vi "PC_Main_SequenceEditor.vi"() -> ()   [LabVIEW 2010]
uses:
  Ctls/StepData.ctl
  <vilib>/Utility/error.llb/DialogType.ctl
  <vilib>/Pansino Software/LabVIEW Architecture/PSARC_Queue Management.llb/PSARC_Queue Create_Single.vi
  <vilib>/Pansino Software/LabVIEW Architecture/PSARC_Queue Management.llb/PSARC_Queue Destroy_Single.vi
  <vilib>/Pansino Software/LabVIEW Architecture/PSARC_Queue Management.llb/PSARC_Queue Valid.vi
  <vilib>/Pansino Software/LabVIEW Architecture/PSARC_Queue Management.llb/PSARC_Queue Insert Element.vi
  <vilib>/Pansino Software/LabVIEW Architecture/PSARC_Queue Management.llb/PSARC_Queue Remove Element.vi
  PC_DynVIs/PC_CallRTGuidedMunitions.vi
panel:
  in  "new element/subarray":T1
  out "Error Report 2":string
  out "Current State 2":string
  in  "TempVariable":T2
  in  "New":bool
  in  "Load":bool
  in  "Save":bool
  in  "Run":bool
  in  "DeleteStep":bool
  in  "EditStep":bool
  in  "AddStep":bool
  in  "Multicolumn Listbox":i32(listbox)
  out "Error Report":string
  out "Current State":string
  in  "OK":bool
  in  "Exit Program":bool
  # "————————————————\nYou could add your temporary variables\nhere.\nThis Control should be saved as a\nvi in your project folder,The proposed vi's block diagram is shown in the picture\n\n\n\n\n\n\n\n————————————————"
  # "/* Path */\nYou could add your path here."
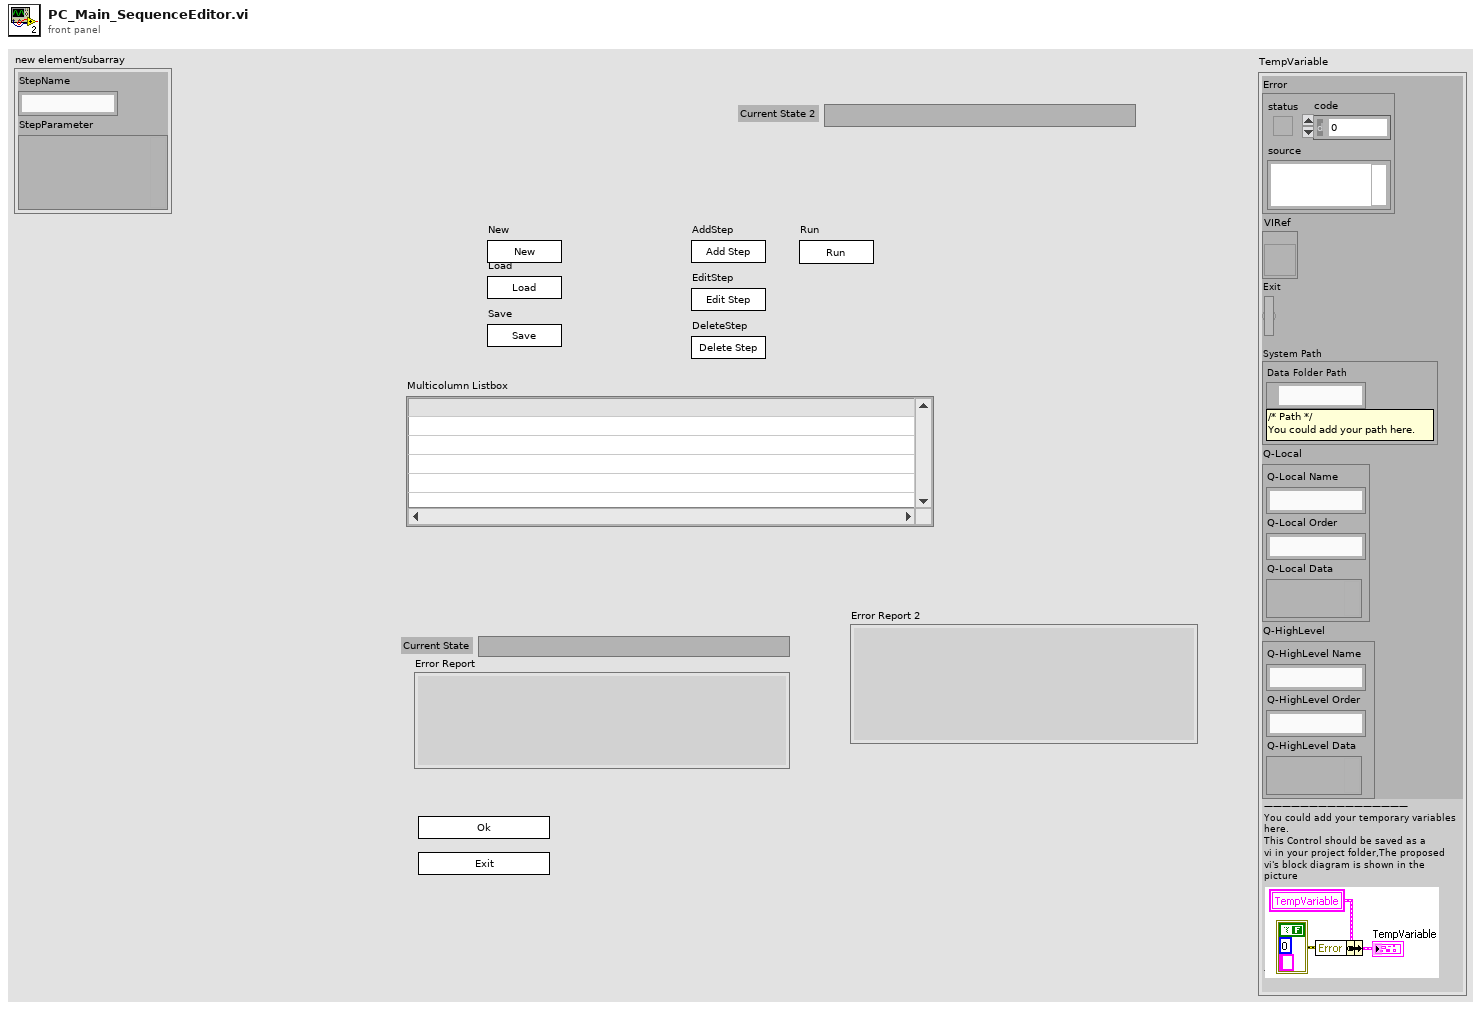
[diagram p1: front panel]
types:
  T1 = typedef "StepData.ctl" = cluster{"StepName":string, "StepParameter":variant}
  T2 = cluster{"Error":errorcluster, "VIRef":refnum<vi>, "Exit":bool, "System Path":cluster{"Data Folder Path":path}, "Q-Local":cluster{"Q-Local Name":string, "Q-Local Order":string, "Q-Local Data":variant}, "Q-HighLevel":cluster{"Q-HighLevel Name":string, "Q-HighLevel Order":string, "Q-HighLevel Data":variant}}
  T3 = typedef "PC_Main_SequenceEditor_TempVariable.ctl" = cluster{"Error":errorcluster, "Event":string, "Data":variant, "VIRef":refnum<vi>, "Exit":bool, "Main Q-Array":string, "Sequence":T1[]}
  T4 = typedef "DialogType.ctl" = u16
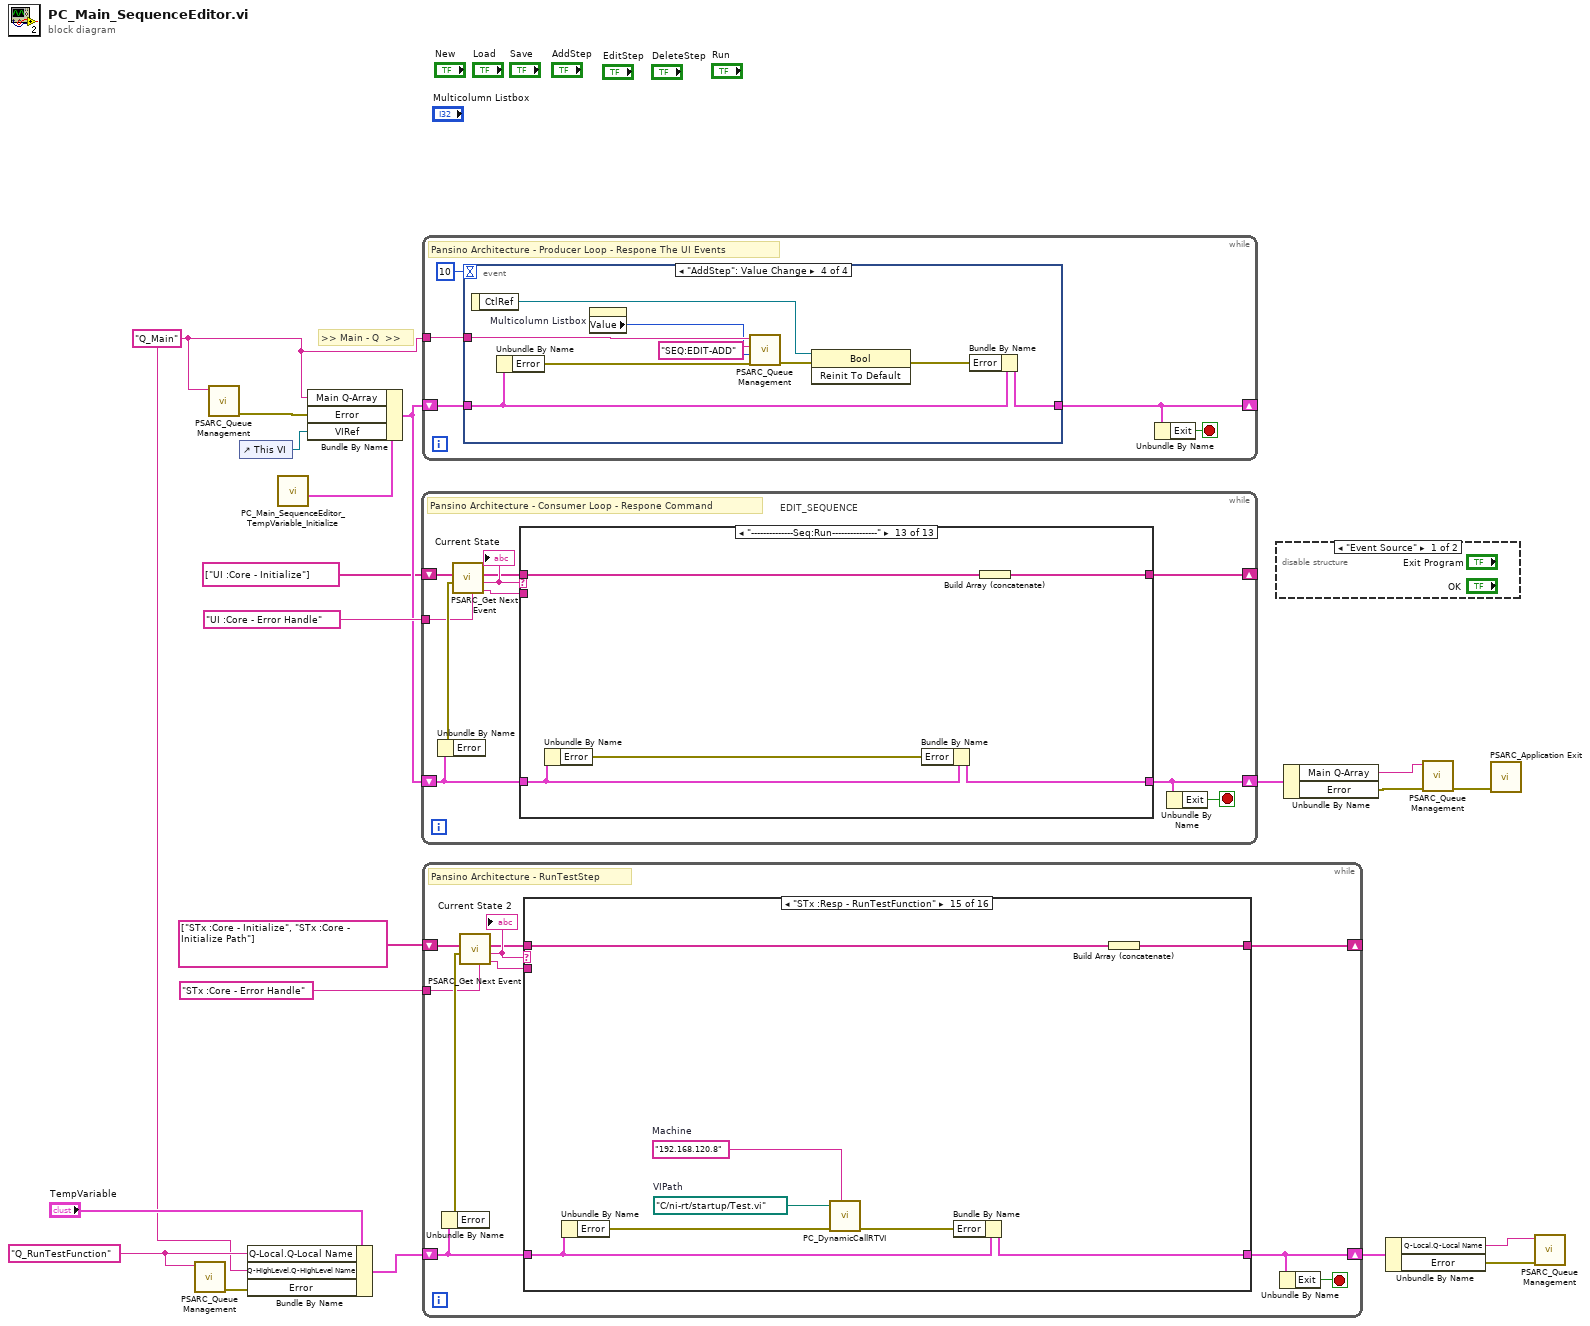
[diagram p0: block diagram]
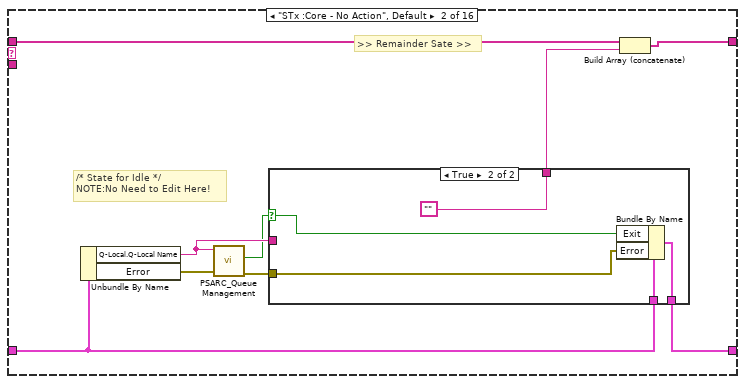
[diagram p3: hidden frame]
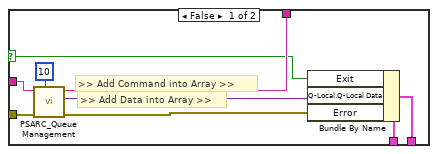
[diagram p4: hidden frame]
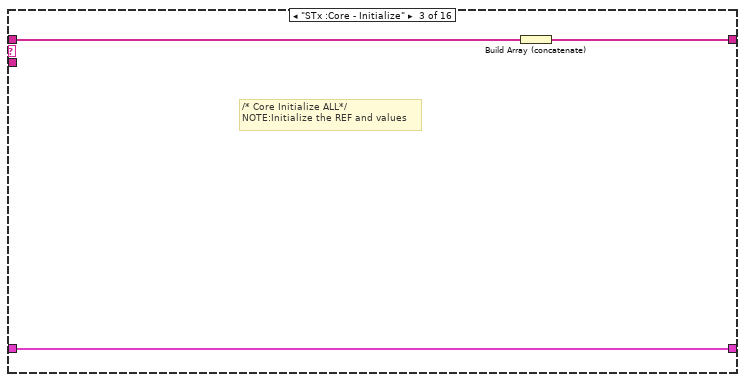
[diagram p5: hidden frame]
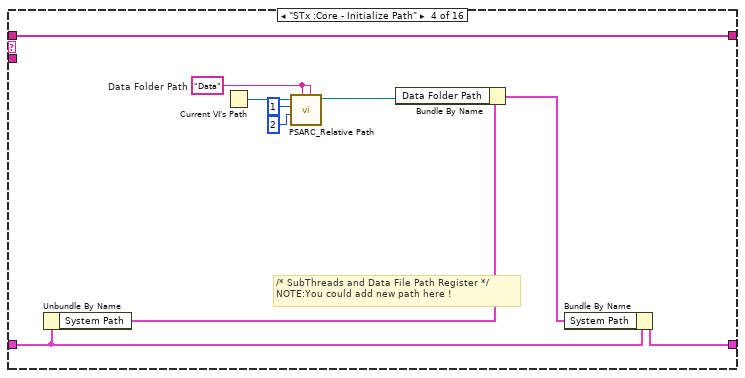
[diagram p6: hidden frame]
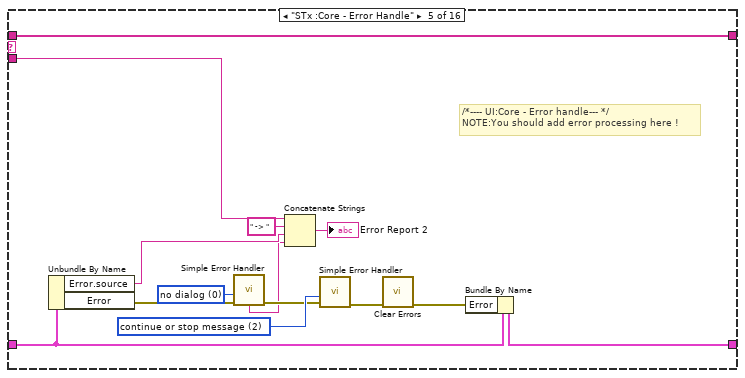
[diagram p7: hidden frame]
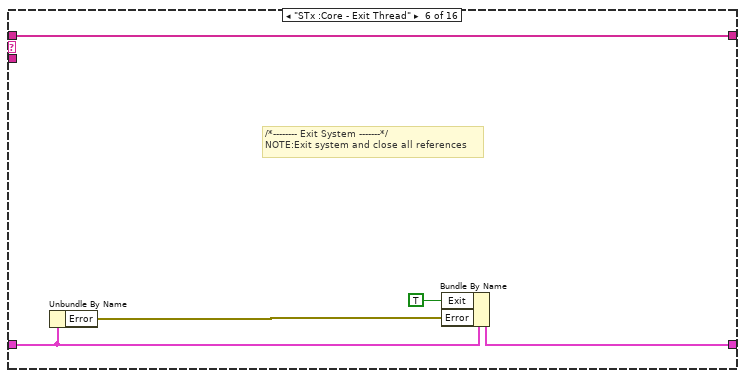
[diagram p8: hidden frame]
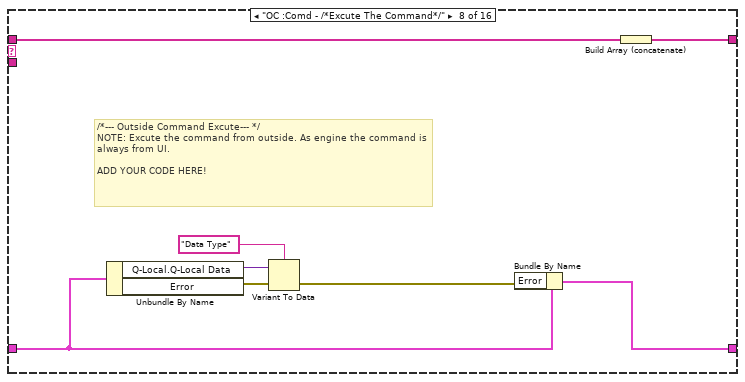
[diagram p10: hidden frame]
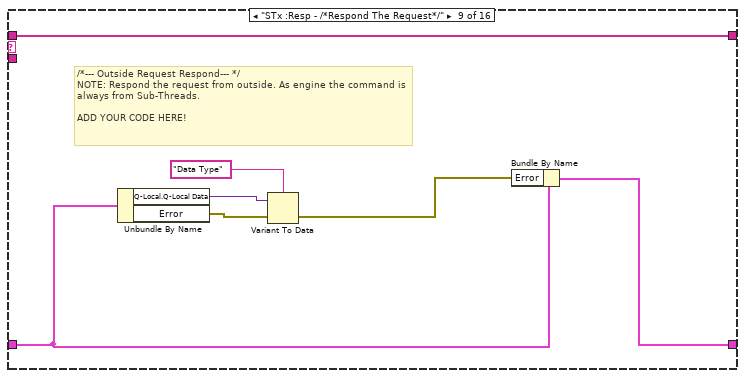
[diagram p11: hidden frame]
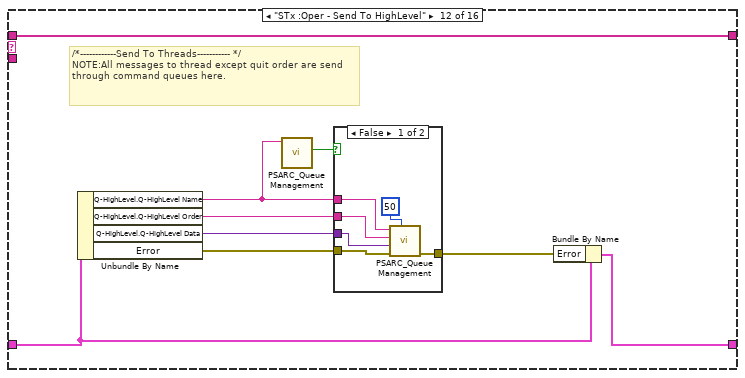
[diagram p14: hidden frame]
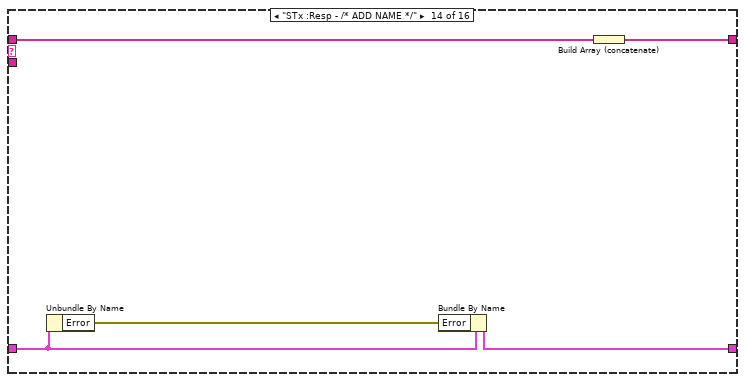
[diagram p17: hidden frame]
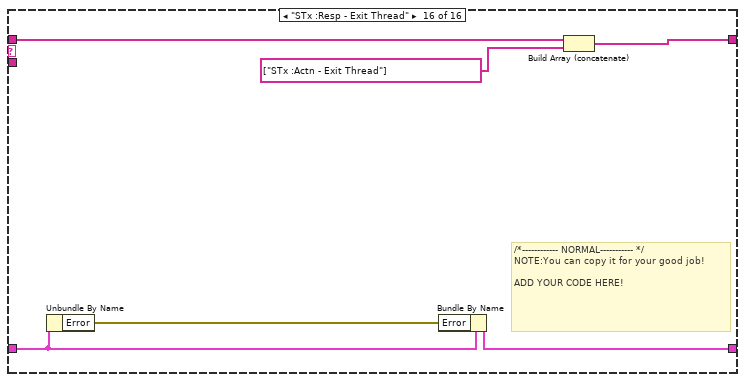
[diagram p18: hidden frame]
diagram:
  w2 = "Q_RunTestFunction" ("Queue Name")
  w1 = "Q_Main" ("Queue name(unamed)")
  # ">> Main - Q  >>"
  n1 = call-poly <vilib>:"PSARC_Queue Management.vi"("Queue Name"=w2) -> ("error out"=w10:errorcluster)  [unwired: 9 in, 1 out]
  n2 = call-poly <vilib>:"PSARC_Queue Management.vi"("Queue Name"=w1) -> ("error out"=w17:errorcluster)  [unwired: 9 in, 1 out]
  n3 = control-ref of="This VI"() -> (w18:refnum<vi>)
  n4 = Bundle By Name(cluster="TempVariable", "Q-Local.Q-Local Name"=w2, "Q-HighLevel.Q-HighLevel Name"=w1, "Error"=w10) -> (w6:T2)
  n5 = call "PC_Main_SequenceEditor_TempVariable_Initialize.vi"() -> ("TempVariable"=w11:T3)  [unwired: 11 in]
  n6 = Bundle By Name(cluster=w11, "Main Q-Array"=w1, "Error"=w17, "VIRef"=w18) -> (w19:T3)
  n7 = while {
    shift-right: [w24] -> w13
    shift-left: w19 -> [w26]
    shift-right: [w27] -> _
    shift-left: string[] ["UI :Core - Initialize"] -> [w30]
    tunnel: "UI :Core - Error Handle" ("Error Handle") -> [w22]
    stop <- w23 stop-if-true
    # "EDIT_SEQUENCE"
    # "Pansino Architecture - Consumer Loop - Respone Command"
    n8 = Unbundle By Name(w26) -> ("Error"=w25:errorcluster)
    n9 = call <vilib>:"PSARC_Get Next Event.vi"("Error Handle"=w22, "error in (no error)"=w25, "event queue in"=w30) -> ("prev event"=w21:string, "next event"=w29:string, "event queue out"=w28:string[])  [unwired: 3 in]
    "Current State" <- w29
    n10 = case shown="\"--------------Seq:Run---------------\"" w29 {
      tunnel: w26 -> [w31 w40 w55 w58 w61 w65 w70 w76 w81 w92 w97 w102 w107]
      tunnel: w28 -> [w32 w38 w57 w59 w64 w66 w68 w74 w79 w90 w95 w100 w105]
      tunnel: [w32 w37 w57 w59 w64 w66 w67 w73 w78 w89 w94 w99 w104] -> w27
      tunnel: [w31 w39 w56 w58 w62 w65 w69 w75 w80 w91 w96 w101 w106] -> w24
      tunnel: w21 -> [_ _ w45 _ _ _ _ _ _ _ _ _ _]
      frame "----------Core Status----------" {
      }
      frame "UI :Core - No Action", Default {
        # "/* State for Idle */\nNo Need to Edit here!"
        # ">> Add Data into the Array >>"
        # ">> Add Command into the Array >>"
        # ">> Remainder Sate >>"
        n11 = Unbundle By Name(w40) -> ("Main Q-Array"=w34:string, "Error"=w41:errorcluster)
        n12 = call-poly <vilib>:"PSARC_Queue Management.vi"("Time out(-1)_queue out"=10, "error in (no error)"=w41, "Queue Name(unamed)"=w34) -> ("error out"=w43:errorcluster, "Data"=w42:variant, "Event"=w35:string)  [unwired: 5 in, 1 out]
        n13 = Wait (ms)(milliseconds to wait=u32 50 ("等待时间（毫秒）")) -> ()  [unwired: 1 out]
        n14 = Bundle By Name(cluster=w40, "Data"=w42, "Error"=w43) -> (w39:T3)
        n15 = Build Array (concatenate)(w38, w35) -> (w37:string[])
      }
      frame "UI :Core - Error Handle" {
        w44 = T4 0 items=["no dialog", "OK message", "continue or stop message", "OK message + warnings", "continue/stop + warnings"] ("type of dialog (OK msg:1)")
        w52 = T4 2 items=["no dialog", "OK message", "continue or stop message", "OK message + warnings", "continue/stop + warnings"] ("type of dialog (OK msg:1)")
        n16 = Unbundle By Name(w55) -> ("Error.source"=w46:string, "Error"=w49:errorcluster)
        n17 = call <vilib>:"Simple Error Handler.vi"("type of dialog (OK msg:1)"=w44, "error in (no error)"=w49) -> ("error out"=w48:errorcluster, "message"=w47:string)  [unwired: 3 in, 3 out]
        n18 = Concatenate Strings(w45, " -> " ("字符串"), w46, w47) -> (→"Error Report":string)
        n19 = call <vilib>:"Simple Error Handler.vi"("type of dialog (OK msg:1)"=w52, "error in (no error)"=w48) -> ("error out"=w54:errorcluster)  [unwired: 3 in, 4 out]
        n20 = call <vilib>:"Clear Errors.vi"("error in (no error)"=w54) -> ("error out"=w53:errorcluster)  [unwired: 6 in]
        n21 = Bundle By Name(cluster=w55, "Error"=w53) -> (w56:T3)
      }
      frame "UI :Core - Initialize" {
        # "/* Resident Queues Register */\nNo Need to Edit here!"
      }
      frame "UI :Core - Exit System" {
        # "/*-------- Exit System -------*/\nExit system and close all references"
        n22 = Unbundle By Name(w61) -> ("Error"=w63:errorcluster)
        n23 = Bundle By Name(cluster=w61, "Exit"=TRUE, "Error"=w63) -> (w62:T3)
      }
      frame "----------Respond Events----------" {
      }
      frame "UI :Resp - /* ADD NAME */" {
        n24 = Unbundle By Name(w70) -> ("Error"=w71:errorcluster)
        n25 = Bundle By Name(cluster=w70, "Error"=w71) -> (w69:T3)
        n26 = Build Array (concatenate)(w68) -> (w67:string[])
      }
      frame "UI :Resp - Exit Event" {
        # "/*------------ NORMAL----------- */\nADD YOUR CODE HERE!\nNOTE:You can copy it for your good job!"
        n27 = Unbundle By Name(w76) -> ("Error"=w77:errorcluster)
        n28 = Bundle By Name(cluster=w76, "Error"=w77) -> (w75:T3)
        n29 = Build Array (concatenate)(w74, string[] ["UI :Core - Exit System"] ("数组")) -> (w73:string[])
      }
      frame "--------------Seq:Edit---------------" {
        n30 = Unbundle By Name(w81) -> ("Error"=w82:errorcluster)
        n31 = Bundle By Name(cluster=w81, "Error"=w82) -> (w80:T3)
        n32 = Build Array (concatenate)(w79) -> (w78:string[])
      }
      frame "SEQ:EDIT-ADD" {
        n33 = Unbundle By Name(w92) -> ("Data"=w84:variant, "Sequence"=w88:T1[], "Error"=w93:errorcluster)
        n34 = Variant To Data(Variant=w84, type=0 ("index")) -> (data=w83:i32)  [unwired: 1 in, 1 out]
        n35 = Insert Into Array(array=w88, index=w83, new element="new element/subarray") -> (w87:T1[])
        n36 = Bundle By Name(cluster=w92, "Sequence"=w87, "Error"=w93) -> (w91:T3)
        n37 = Build Array (concatenate)(w90) -> (w89:string[])
      }
      frame "SEQ:EDIT-EDIT" {
        n38 = Unbundle By Name(w97) -> ("Error"=w98:errorcluster)
        n39 = Bundle By Name(cluster=w97, "Error"=w98) -> (w96:T3)
        n40 = Build Array (concatenate)(w95) -> (w94:string[])
      }
      frame "SEQ:EDIT-DELETE" {
        n41 = Unbundle By Name(w102) -> ("Error"=w103:errorcluster)
        n42 = Bundle By Name(cluster=w102, "Error"=w103) -> (w101:T3)
        n43 = Build Array (concatenate)(w100) -> (w99:string[])
      }
      frame "--------------Seq:Run---------------" {
        n44 = Unbundle By Name(w107) -> ("Error"=w108:errorcluster)
        n45 = Bundle By Name(cluster=w107, "Error"=w108) -> (w106:T3)
        n46 = Build Array (concatenate)(w105) -> (w104:string[])
      }
    }
    n47 = Unbundle By Name(w24) -> ("Exit"=w23:bool)
  }
  n48 = while {
    shift-right: [w111] -> _
    shift-left: w19 -> [w112]
    tunnel: w1 -> [w109]
    stop <- w110 stop-if-true
    # "Pansino Architecture - Producer Loop - Respone The UI Events"
    n49 = event shown="[3] \"AddStep\": Value Change" {
      selector: _ -> [_ _ _ _]
      dyn-events: _ -> [_ _ _ _]
      timeout: 10 -> [_ _ _ _]
      tunnel: w112 -> [w117 w121 w126 w135]
      tunnel: [w116 w120 w125 w134] -> w111
      tunnel: w109 -> [w115 w118 w124 w133]
      event Timeout {
        n50 = event-data() -> ()  [unwired: 1 in, 1 out]
        n51 = call-poly <vilib>:"PSARC_Queue Management.vi"("Queue Name(unamed)"=w115) -> ("Not a queue?"=w114:bool)  [unwired: 9 in, 1 out]
        n52 = Bundle By Name(cluster=w117, "Exit"=w114) -> (w116:T3)
      }
      event "Exit Program": Value Change {
        n53 = event-data() -> ()  [unwired: 1 in, 1 out]
        n54 = Unbundle By Name(w121) -> ("Error"=w122:errorcluster)
        n55 = call-poly <vilib>:"PSARC_Queue Management.vi"("error in (no error)"=w122, "Event"="UI :Resp - Exit Event", "Queue Name(unamed)"=w118) -> ("error out"=w119:errorcluster)  [unwired: 7 in, 1 out]
        n56 = Bundle By Name(cluster=w121, "Error"=w119) -> (w120:T3)
      }
      event "OK": Value Change {
        n57 = event-data() -> ("CtlRef"=w131:refnum<vi>)  [unwired: 1 in]
        n58 = Unbundle By Name(w126) -> ("Error"=w129:errorcluster)
        n59 = call-poly <vilib>:"PSARC_Queue Management.vi"("error in (no error)"=w129, "Event"="UI :Resp - /* ADD NAME */", "Queue Name(unamed)"=w124) -> ("error out"=w128:errorcluster)  [unwired: 7 in, 1 out]
        n60 = invoke class="Bool" method="Reinit To Default"(reference=w131, error in=w128) -> (error out=w127:errorcluster)  [unwired: 1 in, 2 out]
        n61 = Bundle By Name(cluster=w126, "Error"=w127) -> (w125:T3)
      }
      event "AddStep": Value Change {
        n62 = event-data() -> ("CtlRef"=w140:refnum<vi>)  [unwired: 1 in]
        n63 = Unbundle By Name(w135) -> ("Error"=w138:errorcluster)
        n64 = property on="Multicolumn Listbox" class="MCListbox (strict)"() -> ("Value"=w132:i32)  [unwired: 2 in, 2 out]
        n65 = call-poly <vilib>:"PSARC_Queue Management.vi"("error in (no error)"=w138, "Data"=w132, "Event"="SEQ:EDIT-ADD", "Queue Name(unamed)"=w133) -> ("error out"=w137:errorcluster)  [unwired: 6 in, 1 out]
        n66 = invoke class="Bool" method="Reinit To Default"(reference=w140, error in=w137) -> (error out=w136:errorcluster)  [unwired: 1 in, 2 out]
        n67 = Bundle By Name(cluster=w135, "Error"=w136) -> (w134:T3)
      }
    }
    n68 = Unbundle By Name(w111) -> ("Exit"=w110:bool)
  }
  n69 = while {
    shift-right: [w144] -> w9
    shift-left: w6 -> [w146]
    shift-right: [w147] -> _
    shift-left: string[] ["STx :Core - Initialize", "STx :Core - Initialize Path"] -> [w150]
    tunnel: "STx :Core - Error Handle" ("Error Handle") -> [w142]
    stop <- w143 stop-if-true
    # "Pansino Architecture - RunTestStep"
    n70 = Unbundle By Name(w146) -> ("Error"=w145:errorcluster)
    n71 = call <vilib>:"PSARC_Get Next Event.vi"("Error Handle"=w142, "error in (no error)"=w145, "event queue in"=w150) -> ("prev event"=w141:string, "next event"=w149:string, "event queue out"=w148:string[])  [unwired: 3 in]
    "Current State 2" <- w149
    n72 = case shown="\"STx :Resp - RunTestFunction\"" w149 {
      tunnel: w146 -> [w151 w161 w177 w186 w200 w204 w208 w214 w223 w225 w227 w234 w245 w250 w259 w264]
      tunnel: w148 -> [w152 w159 w178 w188 w202 w207 w209 w217 w224 w226 w228 w237 w246 w248 w257 w262]
      tunnel: [w152 w158 w176 w188 w202 w207 w209 w215 w224 w226 w228 w237 w246 w247 w256 w261] -> w147
      tunnel: [w151 w160 w177 w187 w201 w205 w208 w216 w222 w225 w227 w233 w245 w249 w258 w263] -> w144
      tunnel: w141 -> [_ _ _ _ w193 _ _ _ _ _ _ _ _ _ _ _]
      frame "----------Core Status----------" {
        # "/----------* System Core Part *----------/\nNOTE:This part included the normal operations in all programs, such as initial, error handle, exit and so on."
      }
      frame "STx :Core - No Action", Default {
        # "/* State for Idle */\nNOTE:No Need to Edit Here!"
        # ">> Remainder Sate >>"
        n73 = Unbundle By Name(w161) -> ("Q-Local.Q-Local Name"=w156:string, "Error"=w155:errorcluster)
        n74 = call-poly <vilib>:"PSARC_Queue Management.vi"("error in (no error)"=w155, "Queue Name(unamed)"=w156) -> ("error out"=w154:errorcluster, "Not a queue?"=w153:bool)  [unwired: 8 in]
        n75 = case shown="True" w153 {
          selector: w153 -> [w162 w173]
          tunnel: w161 -> [w168 w174]
          tunnel: [w167 w171] -> w160
          tunnel: [w166 "" ("Event")] -> w157
          tunnel: w156 -> [w164 _]
          tunnel: w154 -> [w163 w172]
          frame False {
            # ">> Add Data into Array >>"
            # ">> Add Command into Array >>"
            n76 = call-poly <vilib>:"PSARC_Queue Management.vi"("Time out(-1)_queue out"=10, "error in (no error)"=w163, "Queue Name(unamed)"=w164) -> ("error out"=w170:errorcluster, "Data"=w169:variant, "Event"=w166:string)  [unwired: 5 in, 1 out]
            n77 = Bundle By Name(cluster=w168, "Exit"=w162, "Q-Local.Q-Local Data"=w169, "Error"=w170) -> (w167:T2)
          }
          frame True {
            n78 = Bundle By Name(cluster=w174, "Exit"=w173, "Error"=w172) -> (w171:T2)
          }
        }
        n79 = Build Array (concatenate)(w159, w157) -> (w158:string[])
      }
      frame "STx :Core - Initialize" {
        # "/* Core Initialize ALL*/\nNOTE:Initialize the REF and values"
        n80 = Build Array (concatenate)(w178) -> (w176:string[])
      }
      frame "STx :Core - Initialize Path" {
        w181 = "Data"  # Data Folder Path
        # "/* SubThreads and Data File Path Register */\nNOTE:You could add new path here !"
        n81 = Unbundle By Name(w186) -> ("System Path"=w180:cluster{"Data Folder Path":path})
        n82 = Current VI's Path() -> (path=w182:path)
        n83 = call <vilib>:"PSARC_Relative Path.vi"("Development Relative Path"=w181, "Run Time relative path"=w181, "Run-Time File Depth"=2, "Development File Depth"=1, "Root Path"=w182) -> ("Relative Path"=w185:path)  [unwired: 5 in, 1 out]
        n84 = Bundle By Name(cluster=w180, "Data Folder Path"=w185) -> (w179:cluster{"Data Folder Path":path})
        n85 = Bundle By Name(cluster=w186, "System Path"=w179) -> (w187:T2)
      }
      frame "STx :Core - Error Handle" {
        w194 = T4 0 items=["no dialog", "OK message", "continue or stop message", "OK message + warnings", "continue/stop + warnings"] ("type of dialog (OK msg:1)")
        w197 = T4 2 items=["no dialog", "OK message", "continue or stop message", "OK message + warnings", "continue/stop + warnings"] ("type of dialog (OK msg:1)")
        # "/*---- UI:Core - Error handle--- */\nNOTE:You should add error processing here !"
        n86 = Unbundle By Name(w200) -> ("Error.source"=w191:string, "Error"=w196:errorcluster)
        n87 = call <vilib>:"Simple Error Handler.vi"("type of dialog (OK msg:1)"=w194, "error in (no error)"=w196) -> ("error out"=w195:errorcluster, "message"=w190:string)  [unwired: 3 in, 3 out]
        n88 = Concatenate Strings(w193, " -> " ("字符串"), w191, w190) -> (→"Error Report 2":string)
        n89 = call <vilib>:"Simple Error Handler.vi"("type of dialog (OK msg:1)"=w197, "error in (no error)"=w195) -> ("error out"=w199:errorcluster)  [unwired: 3 in, 4 out]
        n90 = call <vilib>:"Clear Errors.vi"("error in (no error)"=w199) -> ("error out"=w198:errorcluster)  [unwired: 6 in]
        n91 = Bundle By Name(cluster=w200, "Error"=w198) -> (w201:T2)
      }
      frame "STx :Core - Exit Thread" {
        # "/*-------- Exit System -------*/\nNOTE:Exit system and close all references"
        n92 = Unbundle By Name(w204) -> ("Error"=w206:errorcluster)
        n93 = Bundle By Name(cluster=w204, "Exit"=TRUE, "Error"=w206) -> (w205:T2)
      }
      frame "----------Send And Resp----------" {
        # "/----------* Send Order And Respond Part *----------/\nNOTE:This part included the queue operations, which is used to send datas and orders to dynamic threads."
      }
      frame "OC :Comd - /*Excute The Command*/" {
        # "/*--- Outside Command Excute--- */\nNOTE: Excute the command from outside. As engine the command is always from UI.\n\nADD YOUR CODE HERE!"
        n94 = Unbundle By Name(w214) -> ("Q-Local.Q-Local Data"=w213:variant, "Error"=w212:errorcluster)
        n95 = Variant To Data(error in=w212, Variant=w213, type="Data Type" ("Data Type")) -> (error out=w210:errorcluster)  [unwired: 1 out]
        n96 = Bundle By Name(cluster=w214, "Error"=w210) -> (w216:T2)
        n97 = Build Array (concatenate)(w217) -> (w215:string[])
      }
      frame "STx :Resp - /*Respond The Request*/" {
        # "/*--- Outside Request Respond--- */\nNOTE: Respond the request from outside. As engine the command is always from Sub-Threads.\n\nADD YOUR CODE HERE!"
        n98 = Unbundle By Name(w223) -> ("Q-Local.Q-Local Data"=w220:variant, "Error"=w221:errorcluster)
        n99 = Variant To Data(error in=w221, Variant=w220, type="Data Type" ("Data Type")) -> (error out=w219:errorcluster)  [unwired: 1 out]
        n100 = Bundle By Name(cluster=w223, "Error"=w219) -> (w222:T2)
      }
      frame "----------Actions----------" {
        # "/----------* Actions *----------/\nNOTE:This part included the ALL the actions."
      }
      frame "----------Operation----------" {
        # "/----------* Operation Part *----------/\nNOTE:This part included the user operations."
      }
      frame "STx :Oper - Send To HighLevel" {
        # "/*------------Send To Threads----------- */\nNOTE:All messages to thread except quit order are send through command queues here."
        n101 = Unbundle By Name(w234) -> ("Q-HighLevel.Q-HighLevel Name"=w236:string, "Q-HighLevel.Q-HighLevel Order"=w231:string, "Q-HighLevel.Q-HighLevel Data"=w230:variant, "Error"=w235:errorcluster)
        n102 = call-poly <vilib>:"PSARC_Queue Management.vi"("Queue Name(unamed)"=w236) -> ("Not a queue?"=w232:bool)  [unwired: 9 in, 1 out]
        n103 = case shown="False" w232 {
          tunnel: w235 -> [w243 w244]
          tunnel: w236 -> [w241 _]
          tunnel: w231 -> [w239 _]
          tunnel: w230 -> [w240 _]
          tunnel: [w238 w244] -> w229
          frame False {
            n104 = call-poly <vilib>:"PSARC_Queue Management.vi"("Time out(-1)_queue in"=50, "error in (no error)"=w243, "Data"=w240, "Event"=w239, "Queue Name(unamed)"=w241) -> ("error out"=w238:errorcluster)  [unwired: 5 in, 1 out]
          }
          frame True {
          }
        }
        n105 = Bundle By Name(cluster=w234, "Error"=w229) -> (w233:T2)
      }
      frame "----------Respond Events----------" {
        # "/----------* Respond Order Part *----------/\nNOTE:This part included the operations from main queue, which is used to respond the dynamic threads."
      }
      frame "STx :Resp - /* ADD NAME */" {
        n106 = Unbundle By Name(w250) -> ("Error"=w251:errorcluster)
        n107 = Bundle By Name(cluster=w250, "Error"=w251) -> (w249:T2)
        n108 = Build Array (concatenate)(w248) -> (w247:string[])
      }
      frame "STx :Resp - RunTestFunction" {
        w252 = "192.168.120.8"  # Machine
        w253 = path "C:/ni-rt/startup/Test.vi"  # VIPath
        n109 = Unbundle By Name(w259) -> ("Error"=w255:errorcluster)
        n110 = call-poly "PC_DynamicCallRTVI.vi"("Machine"=w252, "error in (no error)"=w255, "VIPath"=w253) -> ("error out"=w254:errorcluster)  [unwired: 7 in, 1 out]
        n111 = Bundle By Name(cluster=w259, "Error"=w254) -> (w258:T2)
        n112 = Build Array (concatenate)(w257) -> (w256:string[])
      }
      frame "STx :Resp - Exit Thread" {
        # "/*------------ NORMAL----------- */\nNOTE:You can copy it for your good job!\n\nADD YOUR CODE HERE!"
        n113 = Unbundle By Name(w264) -> ("Error"=w265:errorcluster)
        n114 = Bundle By Name(cluster=w264, "Error"=w265) -> (w263:T2)
        n115 = Build Array (concatenate)(w262, string[] ["STx :Actn - Exit Thread"] ("数组")) -> (w261:string[])
      }
    }
    n116 = Unbundle By Name(w144) -> ("Exit"=w143:bool)
  }
  n117 = disable-structure shown="\"Event Source\"" {
    frame condition #0 (active) {
    }
    frame condition #1 {
    }
  }
  n118 = Unbundle By Name(w13) -> ("Main Q-Array"=w16:string, "Error"=w14:errorcluster)
  n119 = Unbundle By Name(w9) -> ("Q-Local.Q-Local Name"=w7:string, "Error"=w8:errorcluster)
  n120 = call-poly <vilib>:"PSARC_Queue Management.vi"("error in (no error)"=w14, "Queue Name(unamed)"=w16) -> ("error out"=w12:errorcluster)  [unwired: 7 in, 2 out]
  n121 = call <vilib>:"PSARC_Application Exit.vi"("error in (no error)"=w12) -> ()  [unwired: 10 in, 1 out]
  n122 = call-poly <vilib>:"PSARC_Queue Management.vi"("error in (no error)"=w8, "Queue Name(unamed)"=w7) -> ()  [unwired: 7 in, 3 out]
